vi "dfd_Update M-band Reconstruction State.vi"(8 "state in":cluster{"state ":dbl[]}[](array[cluster]), 9 "number of bands":i32, 10 "coefficients":dbl[](array[numeric]), 11 "x":dbl[][](array[numeric])) -> (0 "state out":cluster{"x 2":dbl[]}[](array[cluster]), 3 "y":dbl[][](array[numeric]))   [LabVIEW 2017, in "NI_DigFilter_FilterBank.lvlib"]
uses:
  <vilib>/addons/Digital Filter Design/NI_DigFilter_FilterBank.lvlib
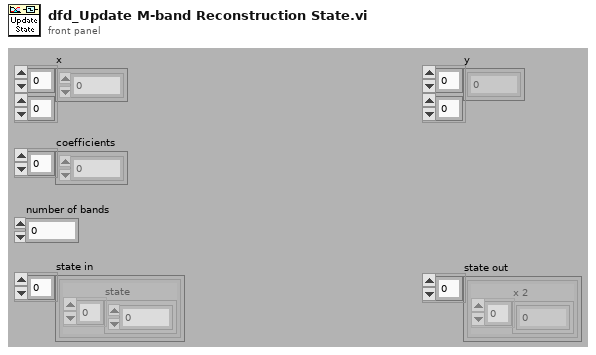
[diagram p1: front panel]
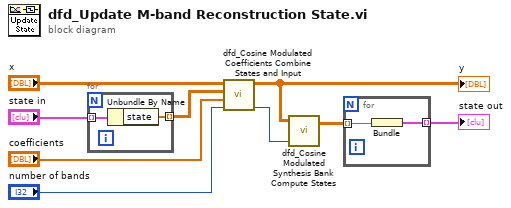
[diagram p0: block diagram]
diagram:
  n1 = for {
    tunnel: [w11] -> w4 mode=indexing
    tunnel: "state in" -> [w10] mode=indexing
    n2 = Unbundle By Name(w10) -> ("state"=w11:dbl[])
  }
  n3 = call <vilib>:"dfd_Cosine Modulated Coefficients Combine States and Input.vi"("number of bands"="number of bands", "coeff"="coefficients", "states in"=w4, "x"="x") -> ("2m-1"=w9:i32, "y"=w1:dbl[][])  [unwired: 6 in]
  "y" <- w1
  n4 = call <vilib>:"dfd_Cosine Modulated Synthesis Bank Compute States.vi"("2m"=w9, "x"=w1) -> ("y"=w2:dbl[][])  [unwired: 2 in]
  n5 = for {
    tunnel: w2 -> [w13] mode=indexing
    tunnel: [w12] -> w6 mode=indexing
    n6 = Bundle("y"=w13) -> (w12:cluster{"y":dbl[]})  [unwired: 1 in]
  }
  "state out" <- w6
